vi "SpaceAvailable.vi"(3 "error in (no error)":errorcluster, 5 "task in":refnum<k24>) -> (0 "error out":errorcluster, 1 "SpaceAvailable":u32, 2 "task out":refnum<k24>)   [LabVIEW 2010]
uses:
  C:/Program Files/National Instruments/LabVIEW 2010/vi.lib/ULx/ULx_LV.dll
  Program Files/National Instruments/LabVIEW 2010/vi.lib/ULx/ULx_LV.dll
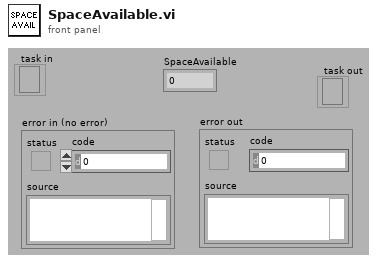
[diagram p1: front panel]
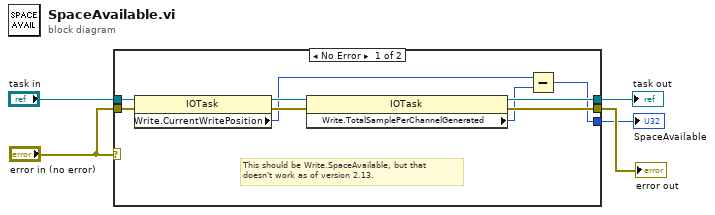
[diagram p0: block diagram]
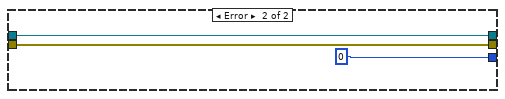
[diagram p2: hidden frame]
diagram:
  n1 = case shown="No Error" "error in (no error)" {
    tunnel: "task in" -> [w14 w17]
    tunnel: "error in (no error)" -> [w13 w16]
    tunnel: [w10 w17] -> w4
    tunnel: [w9 w16] -> w3
    tunnel: [w6 u32 0 ("Read.AvailableSamplePerChannel")] -> w1
    frame No Error {
      # "This should be Write.SpaceAvailable, but that\ndoesn't work as of version 2.13."
      n2 = property class="IOTask"(reference=w14, error in=w13) -> (reference out=w11:refnum<k24>, error out=w12:errorcluster, "Write.CurrentWritePosition"=w8:u32)
      n3 = property class="IOTask"(reference=w11, error in=w12) -> (reference out=w10:refnum<k24>, error out=w9:errorcluster, "Write.TotalSamplePerChannelGenerated"=w7:u32)
      n4 = Subtract(x=w8, y=w7) -> (x-y=w6:u32)
    }
    frame Error {
    }
  }
  "task out" <- w4
  "error out" <- w3
  "SpaceAvailable" <- w1
